vi "cRIO Vision.vi"(0 "address":string="10.8.36.11", 3 "port":u16=10837) -> (12 "Broken":bool, 13 "TurningAngle":sgl, 14 "X":sgl, 15 "Y":sgl, 16 "PrimaryAngle":sgl, 17 "Z":sgl, 18 "ShootingAngle":sgl, 19 "RD":sgl)   [LabVIEW 2012]
uses:
  <vilib>/Utility/error.llb/DialogType.ctl
  Robot Global Data.vi
panel:
  out "Error Count":i32
  out "error out":errorcluster
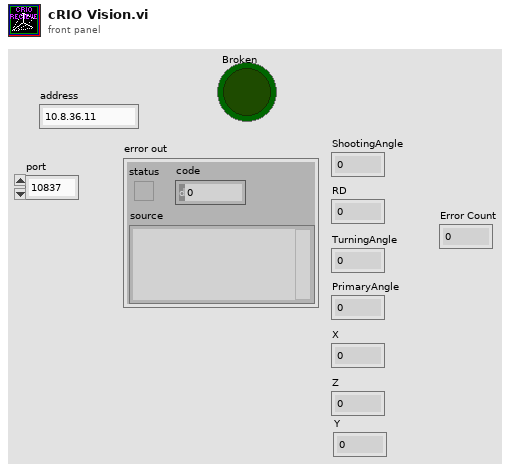
[diagram p1: front panel]
types:
  T1 = enum16{"Standard", "Buffered", "CRLF", "Immediate"}
  T2 = typedef "DialogType.ctl" = u16
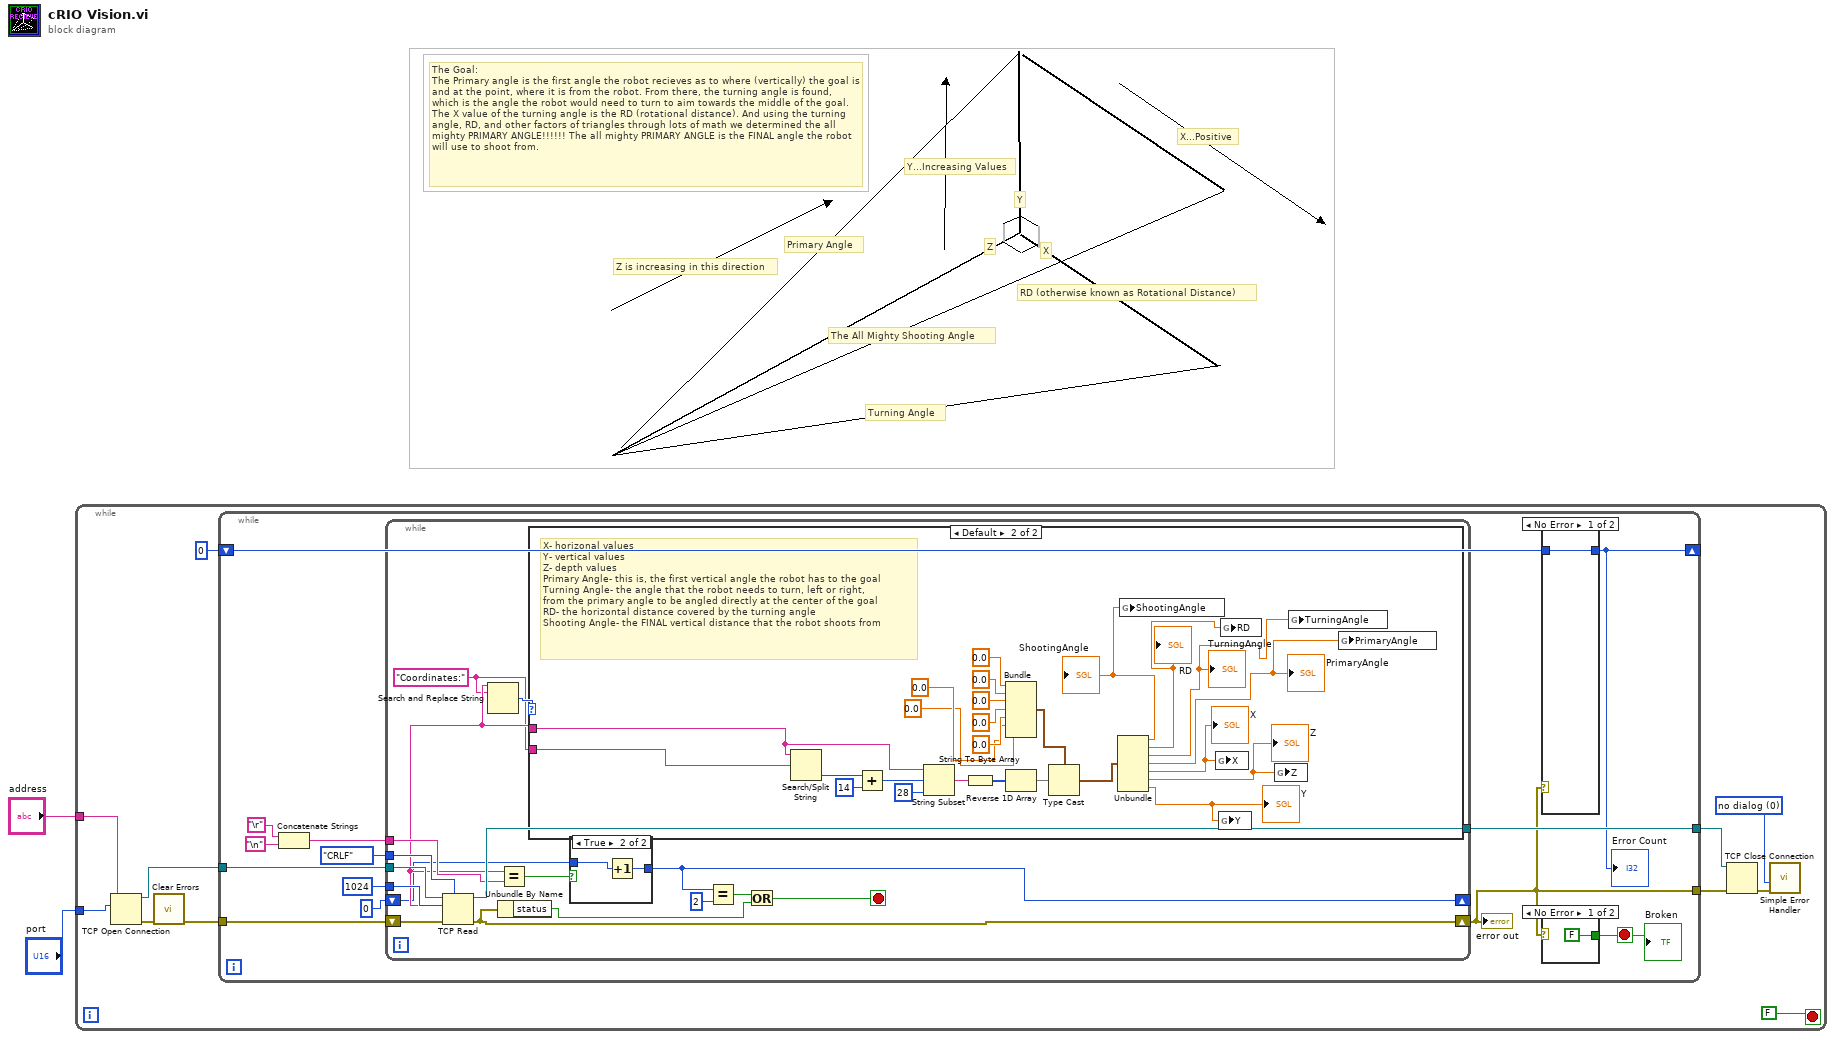
[diagram p0: block diagram]
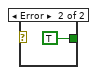
[diagram p2: hidden frame]
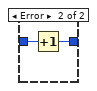
[diagram p3: hidden frame]
diagram:
  # "The Goal:\nThe Primary angle is the first angle the robot recieves as to where (vertically) the goal is and at the point, where it is from the robot. From there, the turning angle is found, which is the angle the robot would need to turn to aim towards the middle of the goal. The X value of the turning angle is the RD (rotational distance). And using the turning angle, RD, and other factors of triangles through lots of math we determined the all mighty PRIMARY ANGLE!!!!!! The all mighty PRIMARY ANGLE is the FINAL angle the robot will use to shoot from."
  # "Z is increasing in this direction"
  # "Y...Increasing Values"
  # "X...Positive"
  # "Z"
  # "Y"
  # "X"
  # "The All Mighty Shooting Angle"
  # "Turning Angle"
  # "Primary Angle"
  # "RD (otherwise known as Rotational Distance)"
  n1 = while {
    tunnel: "port" -> [w13]
    tunnel: "address" -> [w3]
    stop <- FALSE stop-if-true
    w4 = T2 0 items=["no dialog", "OK message", "continue or stop message", "OK message + warnings", "continue/stop + warnings"] ("type of dialog (OK msg:1)")
    n2 = TCP Open Connection(address=w3, remote port or service name=w13) -> (connection ID=w12:refnum<k5>, error out=w11:errorcluster)  [unwired: 3 in]
    n3 = call <vilib>:"Clear Errors.vi"("error in (no error)"=w11) -> ("error out"=w10:errorcluster)  [unwired: 6 in]
    n4 = while {
      tunnel: w12 -> [w16]
      tunnel: w10 -> [w15]
      tunnel: [w21] -> w9
      tunnel: [w14] -> w8
      shift-right: [w18] -> _
      shift-left: 0 -> [w19]
      stop <- w17 stop-if-true
      n5 = Concatenate Strings("\r", "\n") -> (w24:string)
      n6 = while {
        tunnel: w16 -> [w48]
        tunnel: [w47] -> w21
        shift-right: [w45] -> _
        shift-left: 0 -> [w32]
        tunnel: w24 -> [w43]
        tunnel: 1024 ("bytes to read") -> [w36]
        tunnel: T1."CRLF" ("mode (standard)") -> [w42]
        shift-right: [w40] -> w14
        shift-left: w15 -> [w41]
        stop <- w34 stop-if-true
        w33 = "Coordinates:" ("regular expression")
        n7 = TCP Read(connection ID=w48, bytes to read=w36, error in (no error)=w41, 7:w42) -> (connection ID out=w47:refnum<k5>, data out=w35:string, error out=w40:errorcluster)  [unwired: 1 in]
        n8 = Search and Replace String(input string=w35, search string=w33) -> (number of replacements=w39:i32)  [unwired: 2 in, 7 out]
        n9 = Unbundle By Name(w40) -> ("status"=w37:bool)
        n10 = Equal?(x=w35, y=w43) -> (x = y?=w46:bool)
        n11 = case shown="Default" w39 {
          tunnel: w35 -> [_ w70]
          tunnel: w33 -> [_ w69]
          frame 0 {
          }
          frame Default {
            # "X- horizonal values\nY- vertical values\nZ- depth values\nPrimary Angle- this is, the first vertical angle the robot has to the goal\nTurning Angle- the angle that the robot needs to turn, left or right,\nfrom the primary angle to be angled directly at the center of the goal\nRD- the horizontal distance covered by the turning angle\nShooting Angle- the FINAL vertical distance that the robot shoots from"
            n12 = Search/Split String(string=w70, search string/char (-)=w69) -> (offset of match=w68:i32)  [unwired: 1 in, 2 out]
            n13 = Add(x=w68, y=14) -> (x+y=w72:i32)
            n14 = String Subset(string=w70, offset (0)=w72, length (rest)=28 ("length (rest)")) -> (substring=w74:string)
            n15 = String To Byte Array(string=w74) -> (unsigned byte array=w76:u8[])
            n16 = Bundle(sgl 0.0, sgl 0.0, sgl 0.0, sgl 0.0, sgl 0.0, sgl 0.0, sgl 0.0) -> (w62:cluster{sgl, sgl, sgl, sgl, sgl, sgl, sgl})  [unwired: 1 in]
            n17 = Reverse 1D Array(array=w76) -> (reversed array=w75:u8[])
            n18 = Type Cast(type=w62, x=w75) -> (*(type *) &x=w61:cluster{sgl, sgl, sgl, sgl, sgl, sgl, sgl})
            n19 = Unbundle(w61) -> (w58:sgl, w57:sgl, w55:sgl, w56:sgl, w52:sgl, w54:sgl, w53:sgl)
            "ShootingAngle" <- w58
            "RD" <- w57
            "PrimaryAngle" <- w56
            "TurningAngle" <- w55
            "X" <- w52
            "Z" <- w54
            "Y" <- w53
            n20 = global write "Robot Global Data.vi" "ShootingAngle"(w58) -> ()
            n21 = global write "Robot Global Data.vi" "X"(w52) -> ()
            n22 = global write "Robot Global Data.vi" "Y"(w53) -> ()
            n23 = global write "Robot Global Data.vi" "RD"(w57) -> ()
            n24 = global write "Robot Global Data.vi" "Z"(w54) -> ()
            n25 = global write "Robot Global Data.vi" "TurningAngle"(w55) -> ()
            n26 = global write "Robot Global Data.vi" "PrimaryAngle"(w56) -> ()
          }
        }
        n27 = case shown="True" w46 {
          tunnel: w32 -> [w49 w51]
          tunnel: [w49 w50] -> w45
          frame False {
          }
          frame True {
            n28 = Increment(x=w51) -> (x+1=w50:i32)
          }
        }
        n29 = Equal?(x=w45, y=2) -> (x = y?=w38:bool)
        n30 = Or(x=w38, y=w37) -> (x .or. y?=w34:bool)
      }
      "error out" <- w14
      n31 = case shown="No Error" w14 {
        tunnel: w19 -> [w29 w31]
        tunnel: [w29 w30] -> w18
        frame No Error {
        }
        frame Error {
          n32 = Increment(x=w31) -> (x+1=w30:i32)
        }
      }
      "Error Count" <- w18
      n33 = case shown="No Error" w14 {
        tunnel: [FALSE TRUE] -> w17
        frame No Error {
        }
        frame Error {
        }
      }
      "Broken" <- w17
    }
    n34 = TCP Close Connection(connection ID=w9, error in (no error)=w8) -> (error out=w5:errorcluster)  [unwired: 1 in, 1 out]
    n35 = call <vilib>:"Simple Error Handler.vi"("type of dialog (OK msg:1)"=w4, "error in (no error)"=w5) -> ()  [unwired: 3 in, 5 out]
  }
